vi "voltage_range.vi"(8 "error in (no error)":errorcluster, 9 "Channel Select":u32(slide)=1 scale=1.0..2.0, 10 "Voltage":dbl, 11 "VISA In":refnum<visa-resource-name>) -> (0 "error out":errorcluster, 3 "VISA Out":refnum<visa-resource-name>)   [LabVIEW 2011]
panel:
  out "Sent String":string
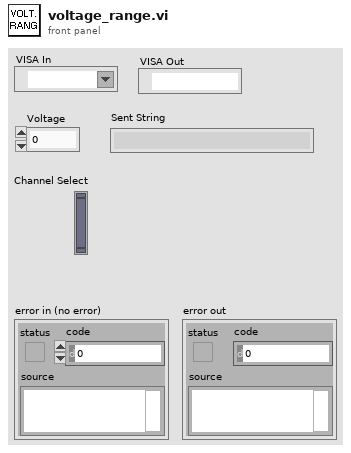
[diagram p1: front panel]
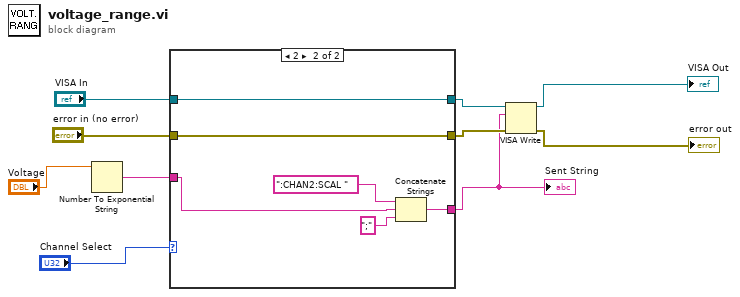
[diagram p0: block diagram]
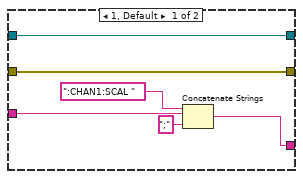
[diagram p2: hidden frame]
diagram:
  n1 = Number To Exponential String(number="Voltage") -> (E-format string=w2:string)  [unwired: 3 in]
  n2 = case shown="2" "Channel Select" {
    tunnel: w2 -> [w13 w19]
    tunnel: [w16 w22] -> w6
    tunnel: "VISA In" -> [w16 w22]
    tunnel: [w15 w21] -> w5
    tunnel: "error in (no error)" -> [w15 w21]
    tunnel: [w11 w17] -> w1
    frame 1, Default {
      n3 = Concatenate Strings(":CHAN1:SCAL " ("string"), w13, ";" ("string")) -> (w11:string)
    }
    frame 2 {
      n4 = Concatenate Strings(":CHAN2:SCAL " ("string"), w19, ";" ("string")) -> (w17:string)
    }
  }
  "Sent String" <- w1
  n5 = VISA Write(VISA resource name=w6, write buffer=w1, error in (no error)=w5) -> (VISA resource name out=→"VISA Out":refnum<visa-resource-name>, error out=→"error out":errorcluster)  [unwired: 1 out]
